vi "Progress Bar Example with User Cancel.vi"() -> ()   [LabVIEW 2015]
uses:
  Library/New Job Status.vi
  Library/New Item Status.vi
  Library/Finish.vi
  Library/Simple Progress Bar.lvlib
panel:
  out "error out":errorcluster
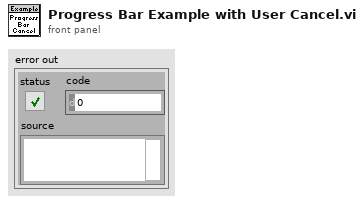
[diagram p1: front panel]
types:
  T1 = typedef "Simple Progress Bar.lvlib/Process Events.ctl" = cluster{"Explorer":refnum<user-event>, "Finished":refnum<user-event>, "Aborted":refnum<user-event>, "New Job":refnum<user-event>, "Item Status":refnum<user-event>, "Item Progression":refnum<user-event>, "Error":refnum<user-event>}
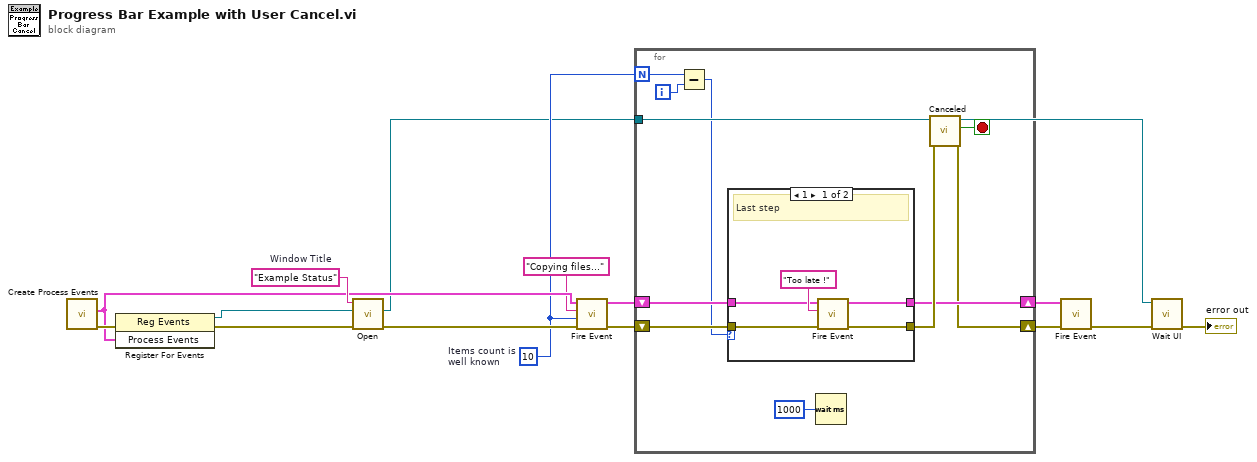
[diagram p0: block diagram]
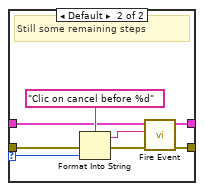
[diagram p2: hidden frame]
diagram:
  w7 = 10  # Items count is  well known
  w12 = "Example Status"  # Window Title
  n1 = call "Create Process Events.vi"() -> ("error out"=w15:errorcluster, "Process Events"=w11:T1)  [unwired: 10 in]
  n2 = register-events(error in=w15, w11) -> (reference out=w13:refnum<event-registration>, error out=w14:errorcluster)  [unwired: 1 in]
  n3 = call "Open.vi"("error in (no error)"=w14, "Process Events Registration"=w13, "Window Title"=w12) -> ("error out"=w10:errorcluster, "UI Events Registration"=w3:refnum<event-registration>)  [unwired: 7 in]
  n4 = call-poly "Fire Event.vi"("error in (no error)"=w10, "Items (unknown)"=w7, "Status"="Copying files...", "Process Events"=w11) -> ("error out"=w8:errorcluster, "Process Events out"=w9:T1)  [unwired: 6 in]
  n5 = for {
    N: w7 -> [w16]
    shift-right: [w18] -> w1
    shift-left: w8 -> [w26]
    shift-right: [w19] -> w2
    shift-left: w9 -> [w23]
    tunnel: w3 -> [w22]
    i -> [w25]
    stop <- w17 stop-if-true
    n6 = Subtract(x=w16, y=w25) -> (x-y=w21:i32)
    n7 = case shown="1" w21 {
      selector: w21 -> [_ w34]
      tunnel: w26 -> [w29 w39]
      tunnel: w23 -> [w30 w36]
      tunnel: [w28 w33] -> w20
      tunnel: [w27 w32] -> w19
      frame 1 {
        # "Last step"
        n8 = call-poly "Fire Event.vi"("error in (no error)"=w29, "Status"="Too late !" ("format string"), "Process Events"=w30) -> ("error out"=w28:errorcluster, "Process Events out"=w27:T1)  [unwired: 7 in]
      }
      frame Default {
        # "Still some remaining steps"
        n9 = Format Into String(format string="Clic on cancel before %d", error in=w39, w34) -> (resulting string=w35:string, error out=w37:errorcluster)  [unwired: 1 in]
        n10 = call-poly "Fire Event.vi"("error in (no error)"=w37, "Status"=w35, "Process Events"=w36) -> ("error out"=w33:errorcluster, "Process Events out"=w32:T1)  [unwired: 7 in]
      }
    }
    n11 = Wait (ms)(milliseconds to wait=u32 1000) -> ()  [unwired: 1 out]
    n12 = call "Canceled.vi"("error in (no error)"=w20, "UI Events Registration"=w22) -> ("error out"=w18:errorcluster, "Canceled by user?"=w17:bool)  [unwired: 8 in]
  }
  n13 = call-poly "Fire Event.vi"("error in (no error)"=w1, "Process Events"=w2) -> ("error out"=w5:errorcluster)  [unwired: 8 in, 1 out]
  n14 = call "Wait UI.vi"("error in (no error)"=w5, "UI Events Registration"=w3) -> ("error out"=→"error out":errorcluster)  [unwired: 7 in, 2 out]
